vi "DSA_computations (subVI).vi"(6 "averaging parameters":T2={"averaging mode"=enum."RMS averaging", "weighting mode"=enum."Exponential", "number of averages"=10.0}, 7 "Restart Averaging":bool, 8 "error in (no error)":errorcluster, 9 "view":cluster{"Channel":u16, "View":u16} {"View" items=["Magnitude", "Phase", "Coherence (FRF only)"]; "Channel" items=["Channel A (stimulus)", "Channel B (response)"]}, 10 "DSA settings":T1={"function"=enum."Frequency response", "baseband span"=20000.0, "window"=enum."Hanning", "resolution (# of lines)"=800}, 11 "stimulus and response":waveform(dbl)[](array[waveform])) -> (0 "error out":errorcluster, 1 "view out":cluster{"Channel":u16, "View":u16} {"View" items=["Magnitude", "Phase", "Coherence (FRF only)"]; "Channel" items=["Channel A (stimulus)", "Channel B (response)"]}, 2 "DSA settings out":T1={"function"=enum."Frequency response", "baseband span"=20000.0, "window"=enum."Hanning", "resolution (# of lines)"=800}, 3 "output array":cluster{"f0":dbl, "df":dbl, "Y":dbl[]}[](array[cluster]))   [LabVIEW 2020]
doc: "This VI encapsulates the different functions used in a DSA instrument.\n<B>Input values : </B>\nStimulus signal \nResponse signal (Output of the Device Under Test)\n\n<B>Returned values : </B>\nWindowed time\nPower spectrum\nFFT (Mag-Phase)\nCross Power Spectrum\nFrequency Response"
uses:
  <vilib>/measure/macond.llb/Scaled Window for 1 Chan.vi
  <vilib>/measure/maspectr.llb/FFT Power Spectrum and PSD for 1 Chan.vi
  <vilib>/measure/maspectr.llb/FFT Spectrum (Mag-Phase) for 1 Chan.vi
  <vilib>/measure/maspectr.llb/Frequency Response Function (Mag-Phase) 1-1.vi
  <vilib>/measure/NI_MAPro.lvlib
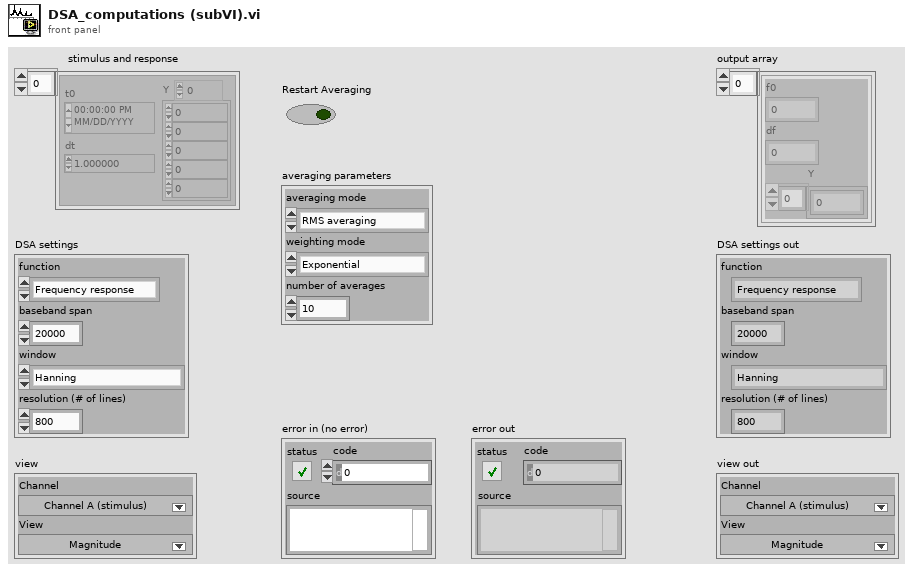
[diagram p1: front panel]
types:
  T1 = cluster{"function":enum16{"Windowed time", "Power Spectrum", "FFT (Mag-Phase)", "Cross Power spectrum", "Frequency response"}, "baseband span":dbl, "window":enum16{"None ", "Hanning", "Hamming", "Blackman-Harris", "Exact Blackman", "Blackman", "Flat Top", "4 Term B-Harris ", "7 Term B-Harris", "Low Sidelobe"}, "resolution (# of lines)":u32}
  T2 = cluster{"averaging mode":enum16{"No averaging", "Vector averaging", "RMS averaging", "Peak hold"}, "weighting mode":enum16{"Linear", "Exponential"}, "number of averages":dbl}
  T3 = cluster{"dB On (F)":bool, "unwrap phase (F)":bool, "convert to degree (F)":bool}
  T4 = enum16{"None ", "Hanning", "Hamming", "Blackman-Harris", "Exact Blackman", "Blackman", "Flat Top", "4 Term B-Harris ", "7 Term B-Harris", "Low Sidelobe"}
  T5 = enum16{"Windowed time", "Power Spectrum", "FFT (Mag-Phase)", "Cross Power spectrum", "Frequency response"}
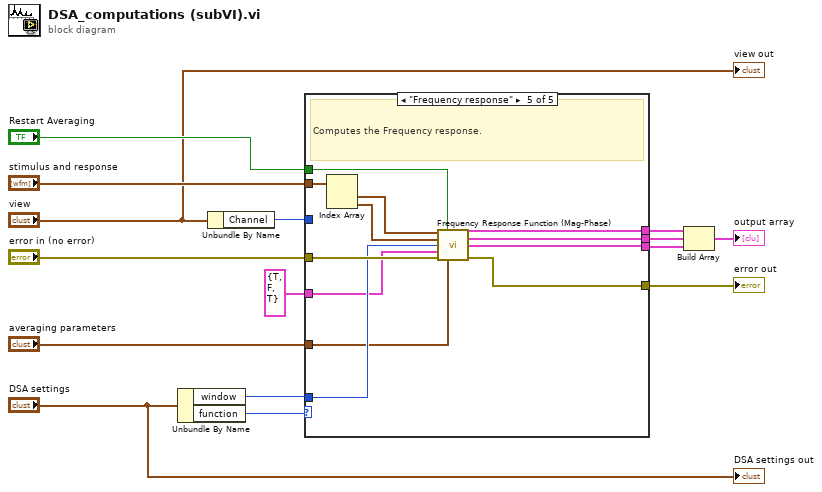
[diagram p0: block diagram]
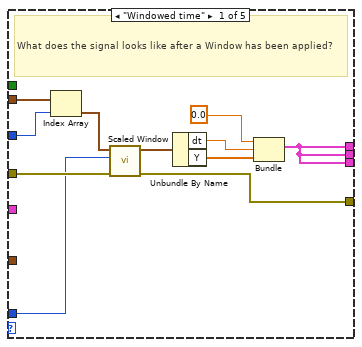
[diagram p2: hidden frame]
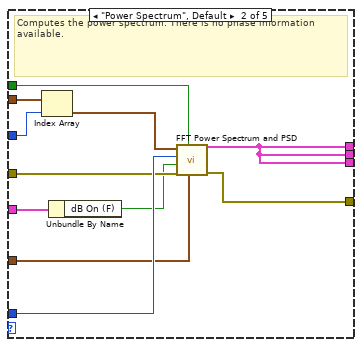
[diagram p3: hidden frame]
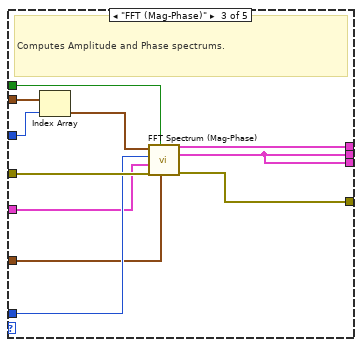
[diagram p4: hidden frame]
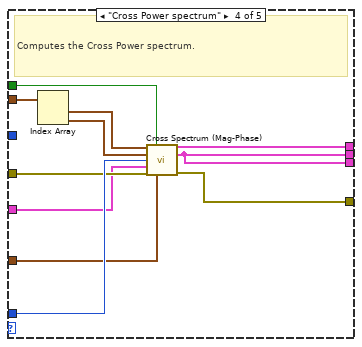
[diagram p5: hidden frame]
diagram:
  n1 = Unbundle By Name("DSA settings") -> ("window"=w9:T4, "function"=w1:T5)
  n2 = Unbundle By Name("view") -> ("Channel"=w7:u16)
  n3 = case shown="\"Frequency response\"" w1 {
    tunnel: "stimulus and response" -> [w26 w37 w48 w59 w71]
    tunnel: w7 -> [w25 w36 w47 _ _]
    tunnel: w9 -> [w22 w34 w44 w56 w67]
    tunnel: "error in (no error)" -> [w23 w33 w45 w54 w70]
    tunnel: [w17 w27 w43 w55 w66] -> w4
    tunnel: [w17 w27 w38 w49 w65] -> w6
    tunnel: "averaging parameters" -> [_ w32 w42 w53 w64]
    tunnel: T3 {"dB On (F)"=TRUE, "unwrap phase (F)"=FALSE, "convert to degree (F)"=TRUE} ("view") -> [_ w31 w41 w52 w63]
    tunnel: "Restart Averaging" -> [_ w29 w40 w51 w62]
    tunnel: [w17 w27 w38 w49 w61] -> w5
    tunnel: [w20 w28 w39 w50 w60] -> w2
    frame "Windowed time" {
      # "What does the signal looks like after a Window has been applied?"
      n4 = Index Array(array=w26, index=w25) -> (element=w24:waveform(dbl))
      n5 = call-poly <vilib>:"Scaled Window.vi"("error in (no error)"=w23, "window"=w22, "signal in"=w24) -> ("error out"=w20:errorcluster, "signal out"=w21:waveform(dbl))  [unwired: 6 in, 1 out]
      n6 = Unbundle By Name(w21) -> ("dt"=w18:dbl, "Y"=w19:dbl[])
      n7 = Bundle(0.0, "dt"=w18, "Y"=w19) -> (w17:cluster{dbl, "dt":dbl, "Y":dbl[]})  [unwired: 1 in]
    }
    frame "Power Spectrum", Default {
      # "Computes the power spectrum. There is no phase information available."
      n8 = Index Array(array=w37, index=w36) -> (element=w35:waveform(dbl))
      n9 = Unbundle By Name(w31) -> ("dB On (F)"=w30:bool)
      n10 = call-poly <vilib>:"FFT Power Spectrum and PSD.vi"("averaging parameters"=w32, "restart averaging (F)"=w29, "error in (no error)"=w33, "dB On (F)"=w30, "window"=w34, "time signal"=w35) -> ("error out"=w28:errorcluster, "Power Spectrum / PSD"=w27:cluster{"f0":dbl, "df":dbl, "magnitude":dbl[]})  [unwired: 2 in, 2 out]
    }
    frame "FFT (Mag-Phase)" {
      # "Computes Amplitude and Phase spectrums."
      n11 = Index Array(array=w48, index=w47) -> (element=w46:waveform(dbl))
      n12 = call-poly <vilib>:"FFT Spectrum (Mag-Phase).vi"("averaging parameters"=w42, "restart averaging (F)"=w40, "error in (no error)"=w45, "view"=w41, "window"=w44, "time signal"=w46) -> ("error out"=w39:errorcluster, "phase"=w38:cluster{"f0":dbl, "df":dbl, "phase":dbl[]}, "magnitude"=w43:cluster{"f0":dbl, "df":dbl, "magnitude":dbl[]})  [unwired: 1 in, 2 out]
    }
    frame "Cross Power spectrum" {
      # "Computes the Cross Power spectrum."
      n13 = Index Array(array=w59) -> (element #1=w58:waveform(dbl), element #2=w57:waveform(dbl))  [unwired: 2 in]
      n14 = call <vilib>:"Cross Spectrum (Mag-Phase).vi"("time signal X"=w58, "restart averaging (F)"=w51, "time signal Y"=w57, "window"=w56, "view"=w52, "error in (no error)"=w54, "averaging parameters"=w53) -> ("magnitude"=w55:cluster{"f0":dbl, "df":dbl, "magnitude":dbl[]}, "phase"=w49:cluster{"f0":dbl, "df":dbl, "phase":dbl[]}, "error out"=w50:errorcluster)  [unwired: 4 in, 2 out]
    }
    frame "Frequency response" {
      # "Computes the Frequency response."
      n15 = Index Array(array=w71) -> (element #1=w69:waveform(dbl), element #2=w68:waveform(dbl))  [unwired: 2 in]
      n16 = call-poly <vilib>:"Frequency Response Function (Mag-Phase).vi"("time signal X"=w69, "restart averaging (F)"=w62, "time signal Y"=w68, "window"=w67, "view"=w63, "error in (no error)"=w70, "averaging parameters"=w64) -> ("magnitude"=w66:cluster{"f0":dbl, "df":dbl, "magnitude":dbl[]}, "phase"=w65:cluster{"f0":dbl, "df":dbl, "phase":dbl[]}, "coherence"=w61:cluster{"f0":dbl, "df":dbl, "coherence":dbl[]}, "error out"=w60:errorcluster)  [unwired: 3 in, 2 out]
    }
  }
  "error out" <- w2
  n17 = Build Array(w4, w6, w5) -> (→"output array":cluster{"f0":dbl, "df":dbl, "coherence":dbl[]}[])
  "view out" <- "view"
  "DSA settings out" <- "DSA settings"
